vi "Thermistor_Manual_Read.vi"(8 "error in":errorcluster, 11 "input cluster":T1={"Core"={"Current VI Reference"=refnum, "Close Panel on Exit?"=FALSE, "Exit"=FALSE, "Initialized?"=FALSE}, "Connections"={"cDAQ DO"={"Task"="", "Connected"=FALSE, "Active"=FALSE, "ID"=""}, "cDAQ AO"={"Task"="", "Connected"=FALSE, "Active"=FALSE, "ID"=""}, "cDAQ AI"={"Task"="", "Connected"=FALSE, "Active"=FALSE, "ID"=""}, "Camera"={"Session"="", "Connected"=FALSE, "Active"=FALSE, "Placeholder"=refnum}, "Humidity"={"Port"="", "Connected"=FALSE, "Active"=FALSE}}, "Data Acquisition"={"Setup"={"Label"="", "Operator"="", "Notes"="", "CircTemp"=1.0, "FlowRate"=1.0}, "Camera"={"Image"=refnum, "Save Image"=refnum, "Image Frequency"=20, "Rectangle"={"Left"=0, "Top"=0, "Right"=0, "Bottom"=0, "Rotation"=0.0}, "Calibration"={"Top Left"={"X"=0.0, "Y"=0.0}, "Top Right"={"X"=0.0, "Y"=0.0}, "Bottom Left"={"X"=0.0, "Y"=0.0}, "Bottom Right"={"X"=0.0, "Y"=0.0}, "Fixpoint"={"X"=0.0, "Y"=0.0}, "Scan Area"=0.0, "Fixpoint Area"=0.0, "Well Pixels"=[], "Valid"=FALSE}, "FocusPos"=0, "Display Mapping"=10}, "Thermistor"={"Sample Size"=1, "Calibration"={"B0.100"=[], "R25"=[], "c"=[], "State"=[], "V_S"=5.0, "R_S"=100.0}, "Timing Mode"=14713}, "Partition"={"Data"=[], "Cell Label"="", "Cell Color"=0, "Height"=10, "Width"=16, "Grid"=[]}, "Queue"={"Queue"=refnum, "Size"=1}, "Sample Rate"=20, "Active"=FALSE, "Ready"=FALSE, "Graph Mode"=0, "Gradient Buffer"=2, "DC Auto"=FALSE}, "Control"={"Sample Rate"=1, "LogStart ms"=0, "AC PSU"={"Voltage"=0.0, "Frequency"=0.0, "State"={"15+16 - Waveform"=0, "17 - Freq Control EN"=FALSE, "18 - Voltage Output"=FALSE, "19 - Output Mode"=0, "20 - Mode Control EN"=FALSE, "21 - AC Control EN"=FALSE, "24 - DC Control EN"=FALSE, "25 - DC Polarity Bias"=FALSE}}, "DC PSU"={"Voltage"=0.0, "Active"=FALSE, "Pulse Size"=0.0, "Pulse Duration"=0.0, "Voltage Set"=0.0}, "Computer Vision"={"Target Pos"=0.0, "Current Pos"=0.0, "Processing"=refnum, "Range"={"Lower value"=128.0, "Upper value"=255.0}, "MinArea"=2, "16-bit Conversion Method"=10, "Display Image"=10, "Binary"=refnum, "Gain"=0.0, "Exposure time"=0.0}, "PID"={"AutoPID"=FALSE, "Gains"={"proportional gain (Kc)"=1.0, "integral time (Ti, min)"=0.01, "derivative time (Td, min)"=0.0}, "autotuning parameters"={"controller type"=1, "relay cycles"=3, "relay amplitude"=1.0, "control specification"=2, "PV noise level"=0.1}, "Show Controls"=FALSE}}, "Manual Temp Control"={"TargetTemp"=1.0, "Mode"=0, "Active"=FALSE}} {"Manual Temp Control"."Mode" items=["Cool", "Heat"]; "Manual Temp Control"."TargetTemp" min=-40.0 max=40.0 step=0.5 format="%#_g °C"; "Control"."PID"."autotuning parameters"."PV noise level" format="%.2f"; "Control"."PID"."autotuning parameters"."control specification" items=["normal", "fast", "slow"]; "Control"."PID"."autotuning parameters"."relay amplitude" format="%.2f"; "Control"."PID"."autotuning parameters"."controller type" items=["PID", "PI", "P"]; "Control"."PID"."Gains"."derivative time (Td, min)" format="%.3f"; "Control"."PID"."Gains"."integral time (Ti, min)" format="%.3f"; "Control"."PID"."Gains"."proportional gain (Kc)" format="%.3f"; "Control"."Computer Vision"."Display Image" items=["Default", "Computer Vision"]; "Control"."Computer Vision"."16-bit Conversion Method" items=["Default"=10, "Most Significant Bits"=11, "Full Dynamic"=12, "Downshift"=13, "Given Range"=14, "90% Dynamic"=15, "Given Percent Range"=16]; "Control"."Computer Vision"."Range"."Upper value" format="%.2f"; "Control"."Computer Vision"."Range"."Lower value" format="%.2f"; "Control"."AC PSU"."State"."19 - Output Mode" items=["Constant Voltage", "Constant Current"]; "Control"."AC PSU"."State"."15+16 - Waveform" items=["Sine", "Square", "Triangle"]; "Control"."Sample Rate" min=1 max=20 step=1 format="%.0f Samples/sec"; "Data Acquisition"."Gradient Buffer" min=2 max=30 step=1; "Data Acquisition"."Graph Mode" items=["Thermistor Temperature", "Camera Temperature"]; "Data Acquisition"."Thermistor"."Timing Mode" items=["Automatic"=16097, "High Resolution"=10195, "High Speed"=14712, "Best 50 Hz Rejection"=14713, "Best 60 Hz Rejection"=14714, "Custom"=10137]; "Data Acquisition"."Thermistor"."Calibration"."R_S" min=0.1 max=1000.0 format="%#_g kOhm"; "Data Acquisition"."Thermistor"."Calibration"."V_S" min=5.0 max=48.0 format="%#_g V"; "Data Acquisition"."Thermistor"."Calibration"."R25" min=0.1 max=1000.0 format="%#_g kOhm"; "Data Acquisition"."Thermistor"."Calibration"."B0.100" min=100.0 max=10000.0 format="%#_g K"; "Data Acquisition"."Thermistor"."Sample Size" min=1 max=200; "Data Acquisition"."Sample Rate" min=20 max=240 format="%.0f samples/min"; "Data Acquisition"."Queue"."Size" min=1 max=200; "Data Acquisition"."Camera"."Display Mapping" items=["Default"=10, "Most Significant Bits"=11, "Full Dynamic"=12, "Downshift"=13, "Given Range"=14, "90% Dynamic"=15, "Given Percent Range"=16]; "Data Acquisition"."Camera"."Calibration"."Fixpoint"."Y" format="%.2f"; "Data Acquisition"."Camera"."Calibration"."Fixpoint"."X" format="%.2f"; "Data Acquisition"."Camera"."Calibration"."Top Left"."Y" format="%.2f"; "Data Acquisition"."Camera"."Calibration"."Top Left"."X" format="%.2f"; "Data Acquisition"."Camera"."Calibration"."Top Right"."Y" format="%.2f"; "Data Acquisition"."Camera"."Calibration"."Top Right"."X" format="%.2f"; "Data Acquisition"."Camera"."Calibration"."Bottom Left"."Y" format="%.2f"; "Data Acquisition"."Camera"."Calibration"."Bottom Left"."X" format="%.2f"; "Data Acquisition"."Camera"."Calibration"."Bottom Right"."Y" format="%.2f"; "Data Acquisition"."Camera"."Calibration"."Bottom Right"."X" format="%.2f"; "Data Acquisition"."Camera"."Rectangle"."Rotation" min=-90.0 max=90.0 step=1.0 format="%.2f"; "Data Acquisition"."Camera"."Rectangle"."Left" scale=0.0..1024.0; "Data Acquisition"."Camera"."Rectangle"."Right" scale=0.0..1024.0; "Data Acquisition"."Camera"."Image Frequency" min=1 max=60 step=1; "Data Acquisition"."Setup"."FlowRate" min=0.0 max=500.0 format="%#_g L/min"; "Data Acquisition"."Setup"."CircTemp" min=-40.0 max=40.0 step=0.5 format="%#_g °C"}) -> (0 "error out":errorcluster, 3 "state":string)   [LabVIEW 2024]
uses:
  DataCluster.ctl
  <vilib>/userDefined/High Color/IMAQdx.ctl
  <vilib>/vision/Image Controls.llb/IMAQ Image.ctl
  DataQueue.ctl
  SensorCluster.ctl
  DataCluster_AC_PSU.ctl
  <vilib>/Platform/TimedLoop/XDataNode/timing_clust.ctl
  <vilib>/Platform/TimedLoop/XDataNode/nitl_modes.ctl
  <vilib>/Platform/TimedLoop/XDataNode/wakeup.ctl
  <extravilib>/ChannelInstances/Tag-bool/Write With Abort.vi
  <extravilib>/ChannelInstances/Tag-bool/Read With Abort.vi
  <extravilib>/ChannelInstances/Tag-bool/Instantiate.vi
  <extravilib>/ChannelInstances/Tag-bool/EndpointRead.vi
  <extravilib>/ChannelInstances/Tag-bool/Endpoint.vi
  <vilib>/platform/TimedLoop/XDataNode/XDataNode.xnode
  <extravilib>/ChannelInstances/Tag-bool.lvlib
  <vilib>/Platform/TimedLoop/XDataNode/XDNodeRunTimeDep.lvlib
panel:
  out "Period (ms)":i64
  in  "Temp/Voltage":enum32{"Temp", "Voltage"}(radio)
  out "T8":dbl format="%.2f °C"
  out "T7":dbl format="%.2f °C"
  out "T6":dbl format="%.2f °C"
  out "T5":dbl format="%.2f °C"
  out "T4":dbl format="%.2f °C"
  out "T3":dbl format="%.2f °C"
  out "T2":dbl format="%.2f °C"
  out "T1":dbl format="%.2f °C"
  out "Status":string
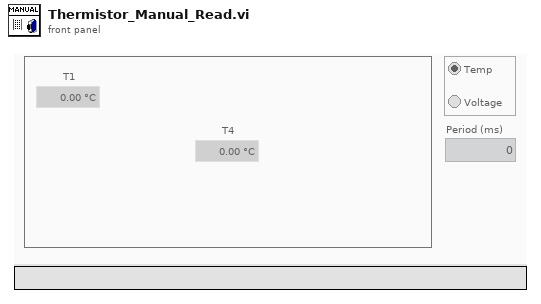
[diagram p1: front panel]
types:
  T1 = typedef "DataCluster.ctl" = cluster{"Core":cluster{"Current VI Reference":refnum<vi>, "Close Panel on Exit?":bool, "Exit":bool, "Initialized?":bool}, "Connections":cluster{"cDAQ DO":cluster{"Task":refnum<k21>, "Connected":bool, "Active":bool, "ID":string}, "cDAQ AO":cluster{"Task":refnum<k21>, "Connected":bool, "Active":bool, "ID":string}, "cDAQ AI":cluster{"Task":refnum<k21>, "Connected":bool, "Active":bool, "ID":string}, "Camera":cluster{"Session":T2, "Connected":bool, "Active":bool, "Placeholder":T3}, "Humidity":cluster{"Port":refnum<visa-resource-name>, "Connected":bool, "Active":bool}}, "Data Acquisition":cluster{"Setup":cluster{"Label":string, "Operator":string, "Notes":string, "CircTemp":dbl, "FlowRate":dbl}, "Camera":cluster{"Image":T3, "Save Image":T3, "Image Frequency":i32, "Rectangle":T4, "Calibration":cluster{"Top Left":T5, "Top Right":T5, "Bottom Left":T5, "Bottom Right":T5, "Fixpoint":T5, "Scan Area":dbl, "Fixpoint Area":dbl, "Well Pixels":cluster{"X":i32, "Y":i32}[][], "Valid":bool}, "FocusPos":u32, "Display Mapping":u32}, "Thermistor":cluster{"Sample Size":i32, "Calibration":cluster{"B0.100":dbl[], "R25":dbl[], "c":dbl[][], "State":bool[], "V_S":dbl, "R_S":dbl}, "Timing Mode":i32}, "Partition":cluster{"Data":string[][], "Cell Label":string, "Cell Color":u32, "Height":i32, "Width":i32, "Grid":string[][]}, "Queue":cluster{"Queue":refnum<queue>, "Size":i32}, "Sample Rate":i32, "Active":bool, "Ready":bool, "Graph Mode":u16, "Gradient Buffer":i32, "DC Auto":bool}, "Control":cluster{"Sample Rate":i32, "LogStart ms":u32, "AC PSU":cluster{"Voltage":dbl[unit], "Frequency":dbl[unit], "State":T6}, "DC PSU":cluster{"Voltage":dbl[unit], "Active":bool, "Pulse Size":dbl[unit], "Pulse Duration":dbl[unit], "Voltage Set":dbl[unit]}, "Computer Vision":cluster{"Target Pos":dbl, "Current Pos":dbl, "Processing":T3, "Range":cluster{"Lower value":sgl, "Upper value":sgl}, "MinArea":i32, "16-bit Conversion Method":u32, "Display Image":u32, "Binary":T3, "Gain":dbl, "Exposure time":dbl}, "PID":cluster{"AutoPID":bool, "Gains":cluster{"proportional gain (Kc)":dbl, "integral time (Ti, min)":dbl, "derivative time (Td, min)":dbl}, "autotuning parameters":cluster{"controller type":u16, "relay cycles":i32, "relay amplitude":dbl, "control specification":u16, "PV noise level":dbl}, "Show Controls":bool}}, "Manual Temp Control":cluster{"TargetTemp":dbl, "Mode":u16, "Active":bool}}
  T2 = typedef "IMAQdx.ctl" = refnum<k21>
  T3 = typedef "IMAQ Image.ctl" = refnum<image>
  T4 = typedef "IMAQ Rectangle" = cluster{"Left":i32, "Top":i32, "Right":i32, "Bottom":i32, "Rotation":dbl}
  T5 = typedef "IMAQ Point" = cluster{"X":sgl, "Y":sgl}
  T6 = typedef "DataCluster_AC_PSU.ctl" = cluster{"15+16 - Waveform":u16, "17 - Freq Control EN":bool, "18 - Voltage Output":bool, "19 - Output Mode":u16, "20 - Mode Control EN":bool, "21 - AC Control EN":bool, "24 - DC Control EN":bool, "25 - DC Polarity Bias":bool}
  T7 = typedef "Tag-bool.lvlib/))Channel.ctl" = refnum<queue>
  T8 = enum8{"Enabled", "Disabled", "Disabled and Grayed Out"}
  T9 = typedef "XDNodeRunTimeDep.lvlib/timing_clust.ctl" = cluster{"Expected End [f-1]":u64, "Actual End [f-1]":u64, "Finished Late? [f-1]":bool, "Expected End [i-1]":u64, "Actual End [i-1]":u64, "Finished Late? [i-1]":bool, "Expected Start [i]":u64, "Actual Start [i]":u64, "Expected Start [f]":u64, "Actual Start [f]":u64, "Source Name":string, "Structure Name":string, "Period":i64, "Deadline":i64, "Offset":i64, "Start":i64, "Priority":i32, "Timeout":i32, "Mode":T10, "Wakeup Reason":T11, "Error":errorcluster, "Source Type":string, "Secondary Source Type":string, "Global End Time":u64, "Global Start Time":u64, "Frame Duration":u64, "Iteration Duration":u64, "Assigned CPU":i32, "I/O Scan Engine Mode":u32}
  T10 = typedef "XDNodeRunTimeDep.lvlib/nitl_modes.ctl" = enum32{"No Change", "Process missed periods, maintain original phase", "Discard missed periods, maintain original phase", "Process missed periods, ignore original phase", "Discard missed periods, ignore original phase"}
  T11 = typedef "XDNodeRunTimeDep.lvlib/wakeup.ctl" = enum32{"Normal", "Aborted", "Asynchronous wakeup", "Timing source error", "Timed loop error", "Timeout"}
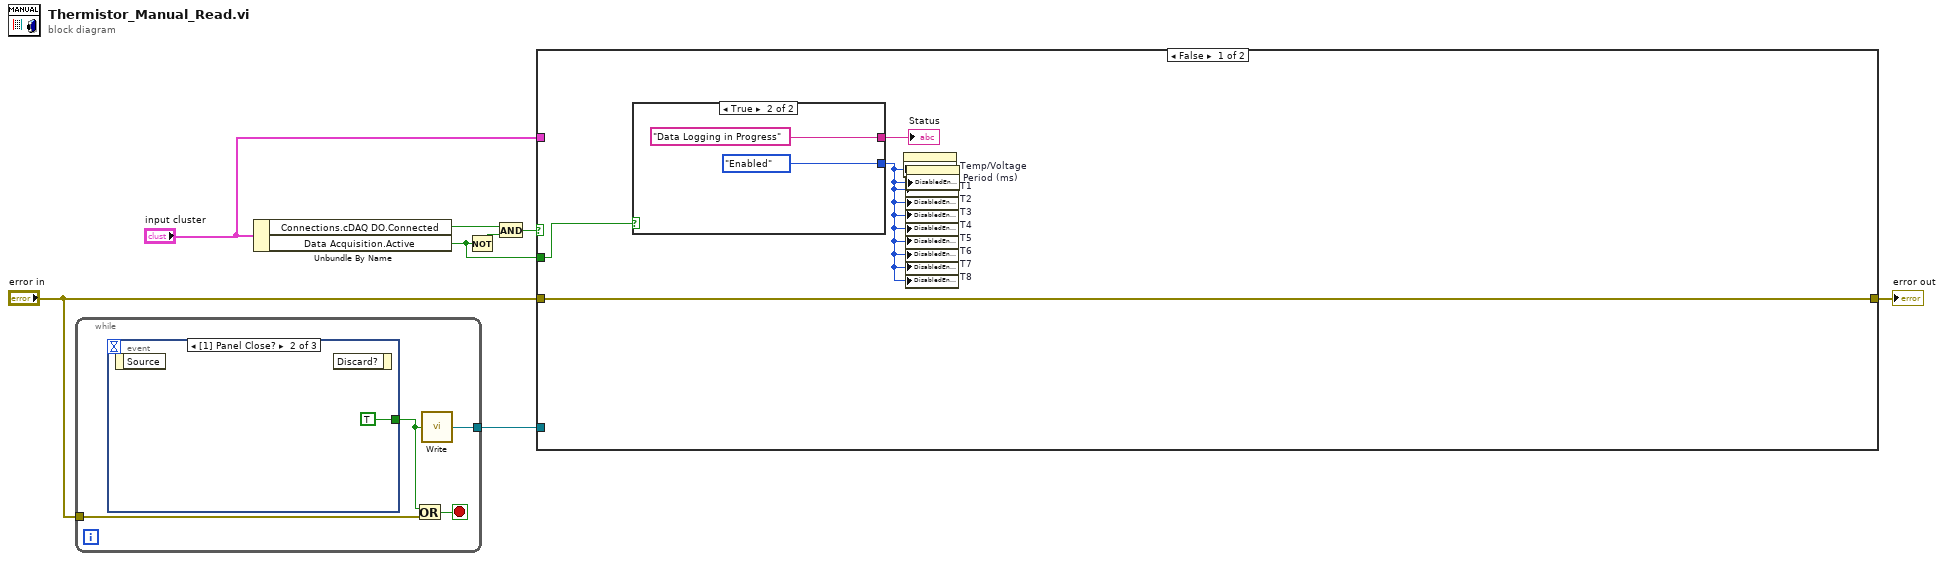
[diagram p0: block diagram]
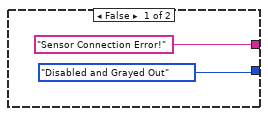
[diagram p2: hidden frame]
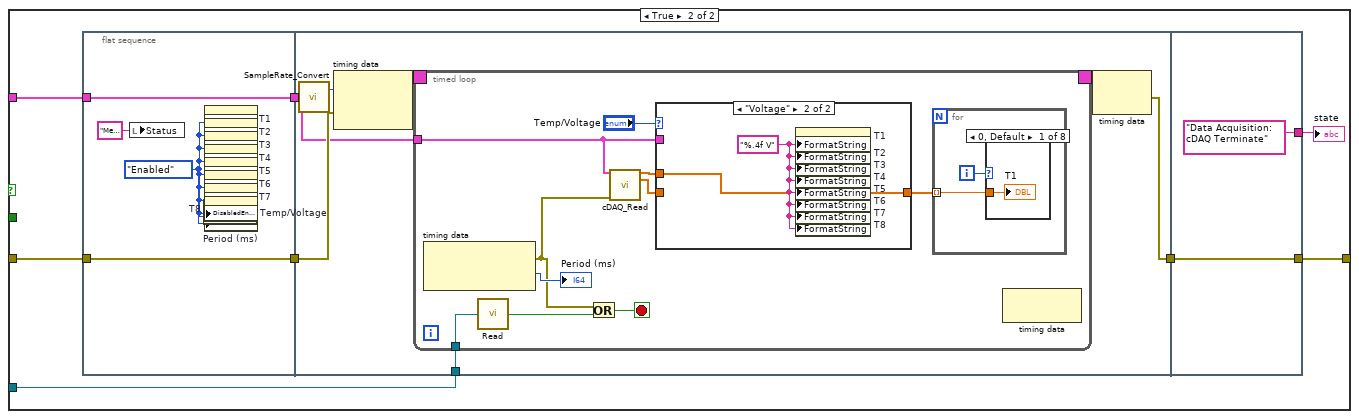
[diagram p3: hidden frame]
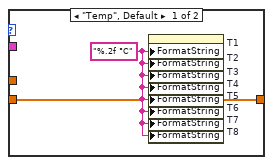
[diagram p4: hidden frame]
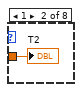
[diagram p5: hidden frame]
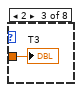
[diagram p6: hidden frame]
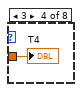
[diagram p7: hidden frame]
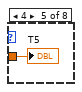
[diagram p8: hidden frame]
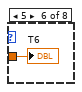
[diagram p9: hidden frame]
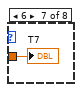
[diagram p10: hidden frame]
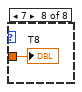
[diagram p11: hidden frame]
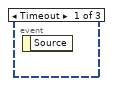
[diagram p12: hidden frame]
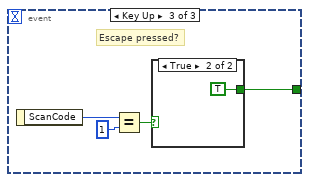
[diagram p13: hidden frame]
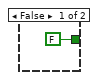
[diagram p14: hidden frame]
diagram:
  n1 = while {
    tunnel: "error in" -> [w10]
    tunnel: [w9] -> w5
    stop <- w11 stop-if-true
    n2 = event shown="[1] Panel Close?" {
      selector: _ -> [_ _ _]
      dyn-events: _ -> [_ _ _]
      timeout: _ -> [_ _ _]
      tunnel: [_ TRUE w17] -> w12
      event Timeout {
        n3 = event-data() -> ()  [unwired: 1 in, 1 out]
      }
      event Panel Close? {
        n4 = event-data() -> ()  [unwired: 1 in, 1 out]
        n5 = event-data() -> ()  [unwired: 2 in, 1 out]
      }
      event Key Up {
        # "Escape pressed?"
        n6 = event-data() -> ("ScanCode"=w16:i16)  [unwired: 1 in]
        n7 = Equal?(x=w16, y=i16 1) -> (x = y?=w14:bool)
        n8 = case shown="True" w14 {
          tunnel: [FALSE TRUE] -> w17
          frame False {
          }
          frame True {
          }
        }
      }
    }
    n9 = Or(x=w12, y=w10) -> (x .or. y?=w11:bool)
    n10 = call <extravilib>:"Write.vi"("element"=w12) -> ("channel"=w9:T7)  [unwired: 1 out]
  }
  n11 = Unbundle By Name("input cluster") -> ("Connections.cDAQ DO.Connected"=w8:bool, "Data Acquisition.Active"=w1:bool)
  n12 = Not(x=w1) -> (.not. x?=w2:bool)
  n13 = And(x=w8, y=w2) -> (x .and. y?=w3:bool)
  n14 = case shown="False" w3 {
    tunnel: "error in" -> [w20 w35]
    tunnel: [w20 w33] -> w7
    tunnel: w5 -> [_ w31]
    tunnel: "input cluster" -> [_ w29]
    tunnel: w1 -> [w21 _]
    frame False {
      n15 = case shown="True" w21 {
        tunnel: ["Sensor Connection Error!" ("String") "Data Logging in Progress" ("String")] -> w23
        tunnel: [T8."Disabled and Grayed Out" ("Disabled") T8."Enabled" ("Disabled")] -> w22
        frame False {
        }
        frame True {
        }
      }
      "Status" <- w23
      n16 = property on="Temp/Voltage" class="RadioBtnsControl (strict)"("DisabledEnum"=w22) -> ()  [unwired: 2 in, 2 out]
      n17 = property on="T1" class="DigNum (strict)"("DisabledEnum"=w22) -> ()  [unwired: 2 in, 2 out]
      n18 = property on="T2" class="DigNum (strict)"("DisabledEnum"=w22) -> ()  [unwired: 2 in, 2 out]
      n19 = property on="T3" class="DigNum (strict)"("DisabledEnum"=w22) -> ()  [unwired: 2 in, 2 out]
      n20 = property on="T4" class="DigNum (strict)"("DisabledEnum"=w22) -> ()  [unwired: 2 in, 2 out]
      n21 = property on="T5" class="DigNum (strict)"("DisabledEnum"=w22) -> ()  [unwired: 2 in, 2 out]
      n22 = property on="T6" class="DigNum (strict)"("DisabledEnum"=w22) -> ()  [unwired: 2 in, 2 out]
      n23 = property on="T7" class="DigNum (strict)"("DisabledEnum"=w22) -> ()  [unwired: 2 in, 2 out]
      n24 = property on="T8" class="DigNum (strict)"("DisabledEnum"=w22) -> ()  [unwired: 2 in, 2 out]
      n25 = property on="Period (ms)" class="DigNum (strict)"("DisabledEnum"=w22) -> ()  [unwired: 2 in, 2 out]
    }
    frame True {
      n26 = flat-sequence {
        tunnel: w35 -> [w36]
        tunnel: [w36] -> w34
        tunnel: [w39] -> w30
        tunnel: w29 -> [w39]
        tunnel: w34 -> [w42]
        tunnel: [w41] -> w32
        tunnel: w31 -> [w46]
        tunnel: w30 -> [w40]
        tunnel: [w81] -> w33
        tunnel: w32 -> [w81]
        tunnel: ["Data Acquisition: cDAQ Terminate"] -> w28
        frame #0 {
          w37 = T8."Enabled" ("Disabled")
          n27 = local write "Status"("Measurement Active!" ("Status")) -> ()
          n28 = property on="Temp/Voltage" class="RadioBtnsControl (strict)"("DisabledEnum"=w37) -> ()  [unwired: 2 in, 2 out]
          n29 = property on="T1" class="DigNum (strict)"("DisabledEnum"=w37) -> ()  [unwired: 2 in, 2 out]
          n30 = property on="T2" class="DigNum (strict)"("DisabledEnum"=w37) -> ()  [unwired: 2 in, 2 out]
          n31 = property on="T3" class="DigNum (strict)"("DisabledEnum"=w37) -> ()  [unwired: 2 in, 2 out]
          n32 = property on="T4" class="DigNum (strict)"("DisabledEnum"=w37) -> ()  [unwired: 2 in, 2 out]
          n33 = property on="T5" class="DigNum (strict)"("DisabledEnum"=w37) -> ()  [unwired: 2 in, 2 out]
          n34 = property on="T6" class="DigNum (strict)"("DisabledEnum"=w37) -> ()  [unwired: 2 in, 2 out]
          n35 = property on="T7" class="DigNum (strict)"("DisabledEnum"=w37) -> ()  [unwired: 2 in, 2 out]
          n36 = property on="T8" class="DigNum (strict)"("DisabledEnum"=w37) -> ()  [unwired: 2 in, 2 out]
          n37 = property on="Period (ms)" class="DigNum (strict)"("DisabledEnum"=w37) -> ()  [unwired: 2 in, 2 out]
        }
        frame #1 {
          n38 = call "SampleRate_Convert.vi"("DataCluster"=w40) -> ("Sample dt (ms)"=w43:i64)  [unwired: 1 out]
          n39 = node-c288(w43, w42) -> (w45:T9)
          n40 = timed-loop {
            tunnel: w46 -> [w55]
            timing: w45 -> [_]
            timing-out: [_] -> w44
            tunnel: w40 -> [w50]
            stop <- w56 stop-if-true
            n41 = node-c288() -> (w47:errorcluster, →"Period (ms)":i64)  [unwired: 1 in]
            n42 = call <extravilib>:"Read.vi"("channel"=w55) -> ("element"=w54:bool)  [unwired: 1 in, 1 out]
            n43 = Or(x=w47, y=w54) -> (x .or. y?=w56:bool)
            n44 = call "cDAQ_Read.vi"("DataCluster"=w50, "error in"=w47) -> ("Voltage Readings"=w48:dbl[], "Temp Readings"=w49:dbl[])  [unwired: 7 in, 5 out]
            n45 = case shown="\"Voltage\"" "Temp/Voltage" {
              tunnel: w49 -> [w61 _]
              tunnel: [w61 w63] -> w52
              tunnel: w50 -> [_ _]
              tunnel: w48 -> [_ w63]
              frame "Temp", Default {
                w62 = "%.2f °C"
                n46 = property on="T1" class="DigNum (strict)"("FormatString"=w62) -> ()  [unwired: 2 in, 2 out]
                n47 = property on="T2" class="DigNum (strict)"("FormatString"=w62) -> ()  [unwired: 2 in, 2 out]
                n48 = property on="T3" class="DigNum (strict)"("FormatString"=w62) -> ()  [unwired: 2 in, 2 out]
                n49 = property on="T4" class="DigNum (strict)"("FormatString"=w62) -> ()  [unwired: 2 in, 2 out]
                n50 = property on="T5" class="DigNum (strict)"("FormatString"=w62) -> ()  [unwired: 2 in, 2 out]
                n51 = property on="T6" class="DigNum (strict)"("FormatString"=w62) -> ()  [unwired: 2 in, 2 out]
                n52 = property on="T7" class="DigNum (strict)"("FormatString"=w62) -> ()  [unwired: 2 in, 2 out]
                n53 = property on="T8" class="DigNum (strict)"("FormatString"=w62) -> ()  [unwired: 2 in, 2 out]
              }
              frame "Voltage" {
                w64 = "%.4f V"
                n54 = property on="T1" class="DigNum (strict)"("FormatString"=w64) -> ()  [unwired: 2 in, 2 out]
                n55 = property on="T2" class="DigNum (strict)"("FormatString"=w64) -> ()  [unwired: 2 in, 2 out]
                n56 = property on="T3" class="DigNum (strict)"("FormatString"=w64) -> ()  [unwired: 2 in, 2 out]
                n57 = property on="T4" class="DigNum (strict)"("FormatString"=w64) -> ()  [unwired: 2 in, 2 out]
                n58 = property on="T5" class="DigNum (strict)"("FormatString"=w64) -> ()  [unwired: 2 in, 2 out]
                n59 = property on="T6" class="DigNum (strict)"("FormatString"=w64) -> ()  [unwired: 2 in, 2 out]
                n60 = property on="T7" class="DigNum (strict)"("FormatString"=w64) -> ()  [unwired: 2 in, 2 out]
                n61 = property on="T8" class="DigNum (strict)"("FormatString"=w64) -> ()  [unwired: 2 in, 2 out]
              }
            }
            n62 = for {
              tunnel: w52 -> [w65] mode=indexing
              i -> [w66]
              n63 = case shown="0, Default" w66 {
                tunnel: w65 -> [w67 w68 w69 w70 w71 w72 w73 w74]
                frame 0, Default {
                  "T1" <- w67
                }
                frame 1 {
                  "T2" <- w68
                }
                frame 2 {
                  "T3" <- w69
                }
                frame 3 {
                  "T4" <- w70
                }
                frame 4 {
                  "T5" <- w71
                }
                frame 5 {
                  "T6" <- w72
                }
                frame 6 {
                  "T7" <- w73
                }
                frame 7 {
                  "T8" <- w74
                }
              }
            }
            n64 = node-c288() -> ()  [unwired: 1 in, 1 out]
          }
          n65 = node-c288(w44) -> (w41:errorcluster)
        }
        frame #2 {
        }
      }
      "state" <- w28
    }
  }
  "error out" <- w7
